vi "Intake_Disc_Set.vi"   [LabVIEW 2018]
uses:
  <vilib>/Rock Robotics/WPI/DriverStation/WPI_DriverStationRobotMode2.ctl
  Intake_Disc_Control_Type.ctl
  Global_Variables/Intake_Disc_Globals.vi
  Global_Variables/Robot_Global_Data.vi
  Global_Variables/Autonomous_Globals.vi
types:
  T1 = typedef "Intake_Disc_Control_Type.ctl" = enum16{"No_Op", "Manual_Disc_Toggle", "Disc_Toggle", "Manual_Press_Toggle", "Press_Toggle", "Acquire_Hatch", "Retract"}
  T2 = typedef "WPI_DriverStationRobotMode2.ctl" = enum16{"Autonomous Disabled", "Autonomous Enabled", "Teleop Disabled", "Teleop Enabled", "Disconnected", "Finish", "Test Disabled", "Test Enabled", "Emergency Stopped"}
  T3 = typedef "Intake_Disc_Notifier.ctl" = cluster{"Intake_Disc_Control_Type":T1, "Manual_Disc_Toggle":bool, "Disc_Toggle":bool, "Disc_Toggle_State":bool, "Manual_Press_Toggle":bool, "Disc_Press_State":bool, "Press_Toggle":bool, "Press_Pnuematic":T4, "Disc_Pnuematic":T4, "Disc_Notifier":refnum<notifier>, "Step":i32}
  T4 = typedef "WPI_SolenoidValue.ctl" = enum16{"Off", "On", "Forward", "Reverse"}
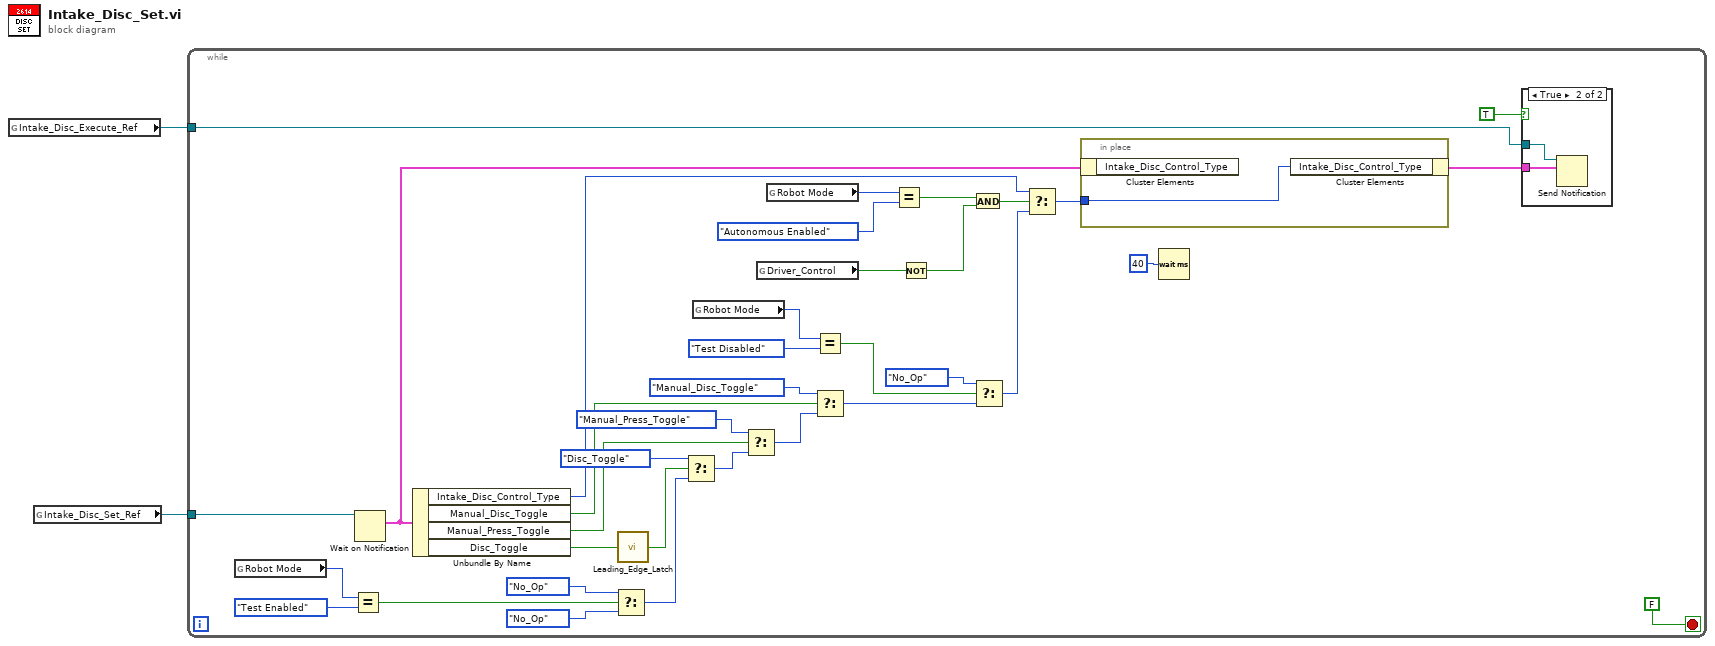
[diagram p0: block diagram]
diagram:
  n1 = global read "Intake_Disc_Globals.vi" "Intake_Disc_Execute_Ref"() -> (w1:refnum<notifier>)
  n2 = global read "Intake_Disc_Globals.vi" "Intake_Disc_Set_Ref"() -> (w2:refnum<notifier>)
  n3 = while {
    tunnel: w2 -> [w36]
    tunnel: w1 -> [w34]
    stop <- FALSE stop-if-true
    n4 = global read "Robot_Global_Data.vi" "Robot Mode"() -> (w28:T2)
    n5 = Equal?(x=w28, y=WPI_DriverStationRobotMode2."Test Enabled") -> (x = y?=w27:bool)
    n6 = Wait on Notification(notifier=w36) -> (notification=w35:T3)  [unwired: 3 in, 3 out]
    n7 = Unbundle By Name(w35) -> ("Intake_Disc_Control_Type"=w30:T1, "Manual_Disc_Toggle"=w23:bool, "Manual_Press_Toggle"=w19:bool, "Disc_Toggle"=w14:bool)
    n8 = Select(t=Intake_Disc_Control_Type."No_Op", s=w27, f=Intake_Disc_Control_Type."No_Op" ("Intake_Disc_Control_Type")) -> (s? t:f=w21:T1)
    n9 = call "Leading_Edge_Latch.vi"("Input"=w14) -> ("Output"=w13:bool)
    n10 = Select(t=Intake_Disc_Control_Type."Disc_Toggle", s=w13, f=w21) -> (s? t:f=w18:T1)
    n11 = global read "Robot_Global_Data.vi" "Robot Mode"() -> (w7:T2)
    n12 = Select(t=Intake_Disc_Control_Type."Manual_Press_Toggle", s=w19, f=w18) -> (s? t:f=w17:T1)
    n13 = global read "Autonomous_Globals.vi" "Driver_Control"() -> (w12:bool)
    n14 = global read "Robot_Global_Data.vi" "Robot Mode"() -> (w32:T2)
    n15 = Equal?(x=w7, y=WPI_DriverStationRobotMode2."Test Disabled") -> (x = y?=w4:bool)
    n16 = Select(t=Intake_Disc_Control_Type."Manual_Disc_Toggle", s=w23, f=w17) -> (s? t:f=w6:T1)
    n17 = Equal?(x=w32, y=WPI_DriverStationRobotMode2."Autonomous Enabled") -> (x = y?=w10:bool)
    n18 = Not(x=w12) -> (.not. x?=w11:bool)
    n19 = And(x=w10, y=w11) -> (x .and. y?=w9:bool)
    n20 = Select(t=Intake_Disc_Control_Type."No_Op", s=w4, f=w6) -> (s? t:f=w5:T1)
    n21 = Select(t=w30, s=w9, f=w5) -> (s? t:f=w33:T1)
    n22 = in-place {
      in-place-border: w33 -> [w41]
      n23 = in-place-cluster #1(w35) -> ()  [unwired: 1 out]
      n24 = in-place-cluster #1("Intake_Disc_Control_Type"=w41) -> (w26:T3)
    }
    n25 = Wait (ms)(milliseconds to wait=u32 40) -> ()  [unwired: 1 out]
    n26 = case shown="True" TRUE {
      tunnel: w34 -> [_ w40]
      tunnel: w26 -> [_ w39]
      frame False {
      }
      frame True {
        n27 = Send Notification(notification=w39, notifier=w40) -> ()  [unwired: 1 in, 2 out]
      }
    }
  }
